vi "FieldOrientedControl.vi"(7 "Orientation Mode":enum16{"Robot-Oriented", "Field-Oriented"}(ring), 8 "Robot_H (deg)":dbl, 10 "Joystick Y":dbl, 11 "Joystick X":dbl) -> (2 "Joystick Y'":dbl, 3 "Joystick X'":dbl)   [LabVIEW 2020]
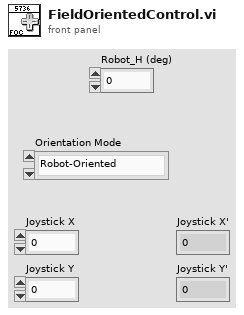
[diagram p1: front panel]
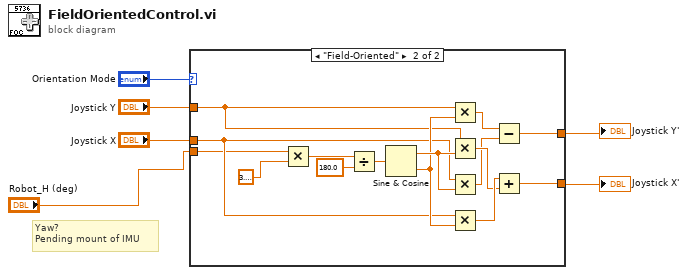
[diagram p0: block diagram]
diagram:
  # "Yaw?\nPending mount of IMU"
  n1 = case shown="\"Field-Oriented\"" "Orientation Mode" {
    tunnel: "Joystick Y" -> [w8 w15]
    tunnel: "Joystick X" -> [w7 w14]
    tunnel: "Robot_H (deg)" -> [_ w12]
    tunnel: [w8 w11] -> w4
    tunnel: [w7 w10] -> w3
    frame "Robot-Oriented", Default {
      # "robot-oriented"
    }
    frame "Field-Oriented" {
      # "field-oriented"
      n2 = Multiply(x=w12, y=3.141592653589793) -> (x*y=w23:dbl)
      n3 = Divide(x=w23, y=180.0) -> (x/y=w22:dbl)
      n4 = Sine & Cosine(0:w22) -> (1:w19:dbl, 2:w18:dbl)
      n5 = Multiply(x=w15, y=w18) -> (x*y=w17:dbl)
      n6 = Multiply(x=w15, y=w19) -> (x*y=w20:dbl)
      n7 = Multiply(x=w14, y=w19) -> (x*y=w16:dbl)
      n8 = Multiply(x=w14, y=w18) -> (x*y=w21:dbl)
      n9 = Subtract(x=w17, y=w16) -> (x-y=w11:dbl)
      n10 = Add(x=w21, y=w20) -> (x+y=w10:dbl)
    }
  }
  "Joystick Y'" <- w4
  "Joystick X'" <- w3
